vi "Builtin.vi"() -> ()   [LabVIEW 2016]
uses:
  <vilib>/Rock Robotics/WPI/Accelerometer/ADXL345 Range.ctl
  <vilib>/Rock Robotics/SystemInterfaces/spilib/spi_bus.ctl
  <vilib>/Rock Robotics/Network Tables/NT Write Numeric Array.vi
  <vilib>/Rock Robotics/WPI/Accelerometer/InternalAccelerometer/WPI_AccelerometerInternalOpen.vi
  <vilib>/Rock Robotics/WPI/Gyro/WPI_GyroAnalogOpen.vi
panel:
  out "Ang Error":dbl
  out "AR Error":dbl
  out "Ang Flutter":dbl
  out "AR Flutter":dbl
  out "Ang Min":dbl
  out "AR Min":dbl
  out "Ang Max":dbl
  out "AR Max":dbl
  out "Angle":dbl
  out "Angular Rate":dbl
  out "Angle":dbl
  out "Calibrated?":bool
  in  "Reset Gyro?":bool
  out "Gyro Found?":bool
  out "Connection Count":i32
  out "Connected":bool
  out "Z Flut":dbl(graph)
  out "Y Flut":dbl(graph)
  out "X Flut":dbl(graph)
  out "Z Accel":dbl(graph)
  out "Y Accel":dbl(graph)
  out "Z Error":dbl
  out "Y Error":dbl
  out "X Error":dbl
  out "X Accel":dbl(graph)
  out "Z Flutter":dbl
  out "Y Flutter":dbl
  out "X Flutter":dbl
  out "X Min":dbl
  out "Y Min":dbl
  out "Z Min":dbl
  out "X Max":dbl
  out "Y Max":dbl
  out "Z Max":dbl
  in  "Accel Range":T1 items=["+/- 2 g", "+/- 4 g", "+/- 8 g", "+/- 16 g"]
  in  "stop":bool
  out "X Acceleration":dbl
  out "Y Acceleration":dbl
  out "Z Acceleration":dbl
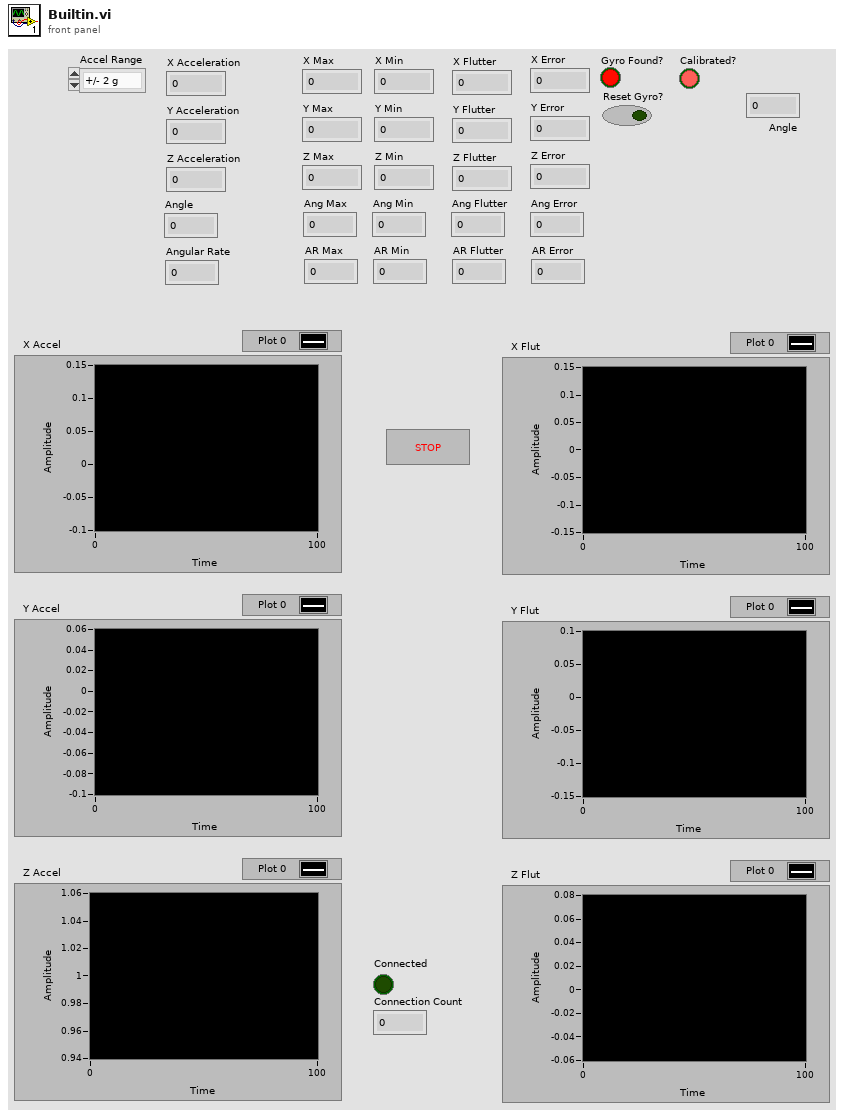
[diagram p1: front panel]
types:
  T1 = typedef "ADXL345 Range.ctl" = u8
  T2 = typedef "spi_bus.ctl" = enum16{"SPI On-Board, CS0", "SPI On-Board, CS1", "SPI On-Board, CS2", "SPI On-Board, CS3", "SPI MXP", "Invalid"}
  T3 = typedef "WPI_GyroDevRef.ctl" = cluster{"DevStatus":errorcluster, "Analog Channel":T4, "Offset":dbl, "Gain (VoltsPerDegree/Second)":dbl, "Gyro Type":enum16{"Analog", "XRS450"}, "Handle":i32, "SPI Bus":T2, "Device Found":bool, "Sample Rate":dbl, "Calibrate On Open":bool}
  T4 = typedef "FPGA_AIChannel.ctl" = enum8{"AI 0", "AI 1", "AI 2", "AI 3", "AI MXP 0", "AI MXP 1", "AI MXP 2", "AI MXP 3", "Invalid"}
  T5 = typedef "WPI_AccelerometerDevRef.ctl" = cluster{"DevStatus":errorcluster, "Scaling":T6, "Analog Channels":T7, "I2C Bus":T8, "SPI Bus":T2, "Accel Range":T1, "ADXL Axes":T9, "Handle":i32, "Device Address":u8, "Accel Type":enum16{"Analog", "ADXL345 I2C", "ADXL345 SPI", "Internal", "ADXL362 SPI"}}
  T6 = typedef "WPI_AccelerometerScaling.ctl" = cluster{"Gain (VoltsPerG)":dbl, "Center Voltage":dbl}
  T7 = typedef "WPI_AccelerometerAnalogChannels.ctl" = cluster{"X-Axis":T4, "Y-Axis":T4, "Z-Axis":T4}
  T8 = typedef "i2c_bus.ctl" = enum16{"I2C On-Board", "I2C MXP", "Invalid"}
  T9 = typedef "WPI_AccelerometerADXL345 Axes.ctl" = cluster{"X-Axis":bool, "Y-Axis":bool, "Z-Axis":bool}
  T10 = cluster{"X-Axis":dbl, "Y-Axis":dbl, "Z-Axis":dbl}
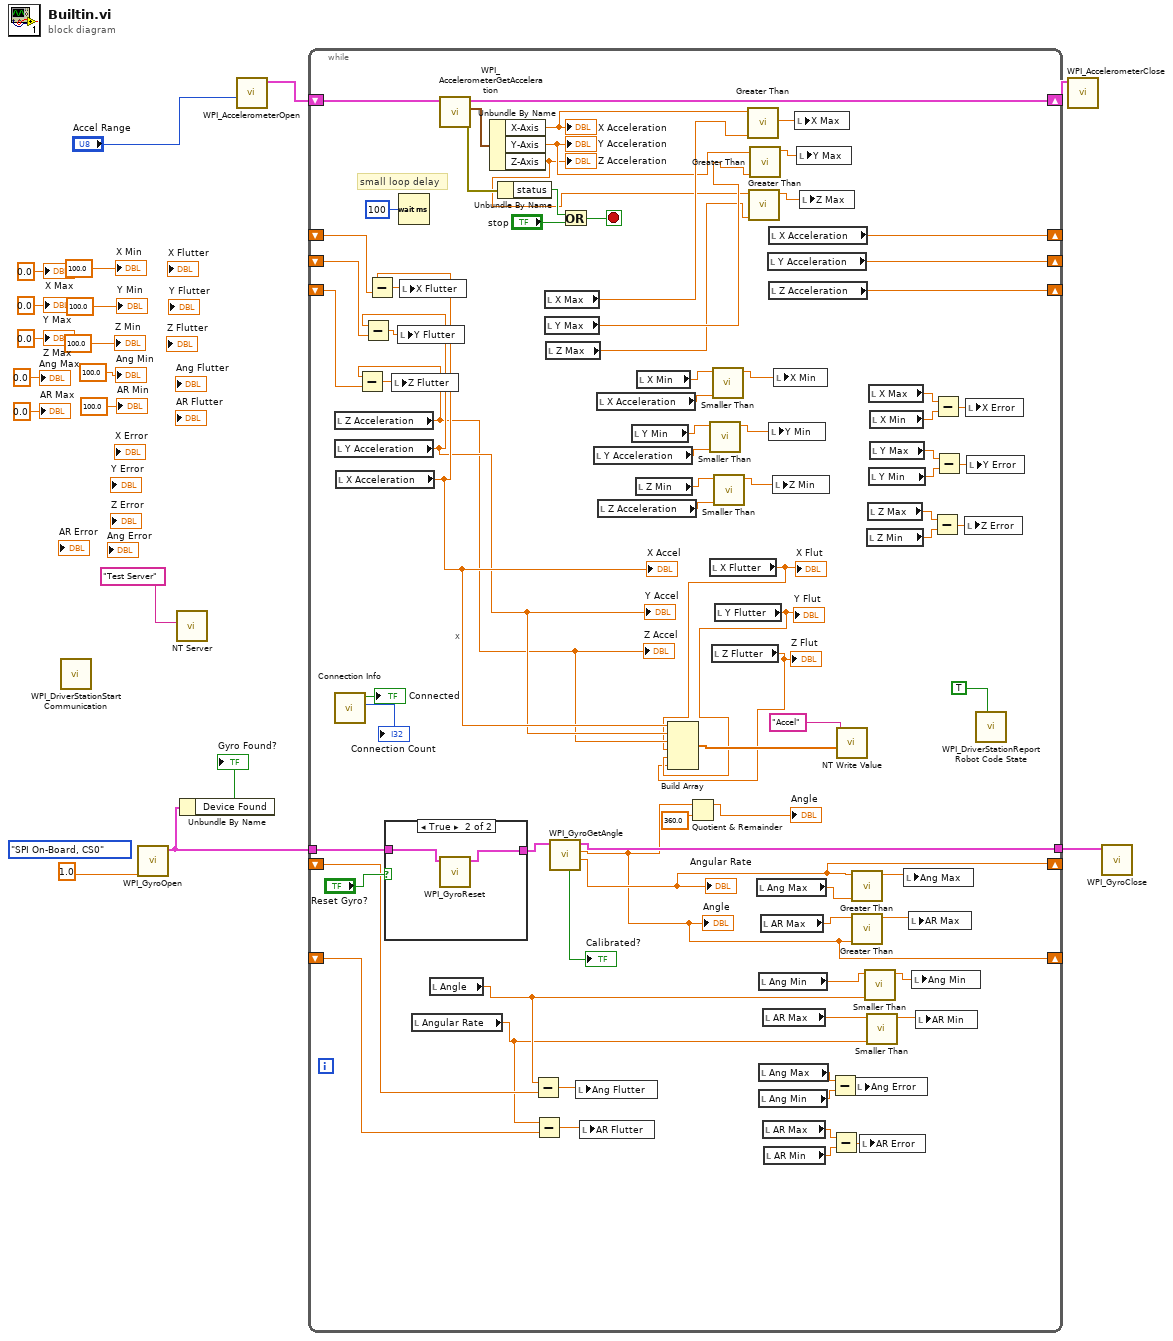
[diagram p0: block diagram]
diagram:
  (unwired) spi_bus."SPI On-Board, CS0" ("SPI Bus")
  n1 = call <vilib>:"WPI_DriverStationStart Communication.vi"() -> ()  [unwired: 12 in]
  n2 = call-poly <vilib>:"WPI_GyroOpen.vi"("Analog Channel"=1.0 ("Sample Rate (ms)")) -> ("GyroDevRef"=w6:T3)  [unwired: 8 in, 2 out]
  n3 = call <vilib>:"NT Server.vi"("Server Name"="Test Server") -> ()  [unwired: 11 in]
  n4 = Unbundle By Name(w6) -> ("Device Found"=→"Gyro Found?":bool)
  n5 = call-poly <vilib>:"WPI_AccelerometerOpen.vi"("Accel Range"="Accel Range") -> ("AccelerometerDevRef"=w18:T5)  [unwired: 9 in, 1 out]
  n6 = while {
    shift-right: [w98] -> w16
    shift-left: w18 -> [w96]
    shift-right: [w76] -> _
    shift-left: _ -> [w71]
    shift-right: [w75] -> _
    shift-left: _ -> [w72]
    shift-right: [w74] -> _
    shift-left: _ -> [w73]
    tunnel: w6 -> [w46]
    tunnel: [w44] -> w5
    shift-right: [w37] -> _
    shift-left: _ -> [w31]
    shift-right: [w36] -> _
    shift-left: _ -> [w27]
    stop <- w97 stop-if-true
    # "X"
    # "small loop delay"
    n7 = local read "Z Acceleration"() -> (w52:dbl)
    "Z Accel" <- w52
    n8 = local read "Y Acceleration"() -> (w53:dbl)
    "Y Accel" <- w53
    n9 = call <vilib>:"Connection Info.vi"() -> ("Connection Count"=→"Connection Count":i32, "Connected"=→"Connected":bool)  [unwired: 10 in]
    n10 = local read "X Acceleration"() -> (w54:dbl)
    "X Accel" <- w54
    n11 = Subtract(x=w52, y=w73) -> (x-y=w68:dbl)
    n12 = Subtract(x=w53, y=w72) -> (x-y=w69:dbl)
    n13 = Subtract(x=w54, y=w71) -> (x-y=w70:dbl)
    n14 = case shown="True" "Reset Gyro?" {
      tunnel: w46 -> [w103 w105]
      tunnel: [w103 w104] -> w45
      frame False {
      }
      frame True {
        n15 = call <vilib>:"WPI_GyroReset.vi"("GyroDevRef"=w105) -> ("GyroDevRef"=w104:T3)  [unwired: 9 in, 1 out]
      }
    }
    n16 = local write "Z Flutter"(w68) -> ()
    n17 = local write "Y Flutter"(w69) -> ()
    n18 = Wait (ms)(milliseconds to wait=u32 100) -> ()  [unwired: 1 out]
    n19 = local write "X Flutter"(w70) -> ()
    n20 = local read "Angular Rate"() -> (w26:dbl)
    n21 = local read "Angle"() -> (w30:dbl)
    n22 = call <vilib>:"WPI_AccelerometerGetAcceleration.vi"("AccelerometerDevRef"=w96) -> ("error out"=w95:errorcluster, "Accelerations"=w99:T10, "AccelerometerDevRef"=w98:T5)  [unwired: 8 in]
    n23 = Unbundle By Name(w99) -> ("X-Axis"=w94:dbl, "Y-Axis"=w91:dbl, "Z-Axis"=w88:dbl)
    "X Acceleration" <- w94
    "Y Acceleration" <- w91
    "Z Acceleration" <- w88
    n24 = Unbundle By Name(w95) -> ("status"=w102:bool)
    n25 = Subtract(x=w30, y=w31) -> (x-y=w29:dbl)
    n26 = Subtract(x=w26, y=w27) -> (x-y=w28:dbl)
    n27 = local read "X Max"() -> (w93:dbl)
    n28 = local read "Y Max"() -> (w90:dbl)
    n29 = local read "Z Max"() -> (w87:dbl)
    n30 = call <vilib>:"WPI_GyroGetAngle.vi"("GyroDevRef"=w45) -> ("Angular Rate"=w37:dbl, "Angle"=w36:dbl, "GyroDevRef"=w44:T3, "Calibrated?"=→"Calibrated?":bool)  [unwired: 6 in, 1 out]
    "Angular Rate" <- w37
    "Angle" <- w36
    n31 = Or(x=w102, y="stop") -> (x .or. y?=w97:bool)
    n32 = local write "Ang Flutter"(w29) -> ()
    n33 = local write "AR Flutter"(w28) -> ()
    n34 = local read "Y Acceleration"() -> (w82:dbl)
    n35 = local read "X Acceleration"() -> (w83:dbl)
    n36 = local read "Z Acceleration"() -> (w77:dbl)
    n37 = local read "Y Min"() -> (w81:dbl)
    n38 = local read "Z Min"() -> (w78:dbl)
    n39 = local read "X Min"() -> (w84:dbl)
    n40 = Quotient & Remainder(x=w36, y=360.0) -> (x-y*floor(x/y)=→"Angle":dbl)  [unwired: 1 out]
    n41 = call "Smaller Than.vi"("N2"=w82, "N1"=w81) -> ("Smaller Number"=w80:dbl)  [unwired: 9 in]
    n42 = local read "X Flutter"() -> (w50:dbl)
    "X Flut" <- w50
    n43 = local read "Z Flutter"() -> (w48:dbl)
    "Z Flut" <- w48
    n44 = call "Smaller Than.vi"("N2"=w83, "N1"=w84) -> ("Smaller Number"=w85:dbl)  [unwired: 9 in]
    n45 = call "Smaller Than.vi"("N2"=w77, "N1"=w78) -> ("Smaller Number"=w79:dbl)  [unwired: 9 in]
    n46 = local read "Y Flutter"() -> (w49:dbl)
    "Y Flut" <- w49
    n47 = Build Array(w54, w53, w52, w50, w49, w48) -> (w51:dbl[])
    n48 = call "Greater Than.vi"("N2"=w93, "N1"=w94) -> ("Greater  Number"=w92:dbl)  [unwired: 9 in]
    n49 = call "Greater Than.vi"("N2"=w87, "N1"=w88) -> ("Greater  Number"=w86:dbl)  [unwired: 9 in]
    n50 = call "Greater Than.vi"("N2"=w90, "N1"=w91) -> ("Greater  Number"=w89:dbl)  [unwired: 9 in]
    n51 = local read "Ang Max"() -> (w41:dbl)
    n52 = local read "Ang Min"() -> (w35:dbl)
    n53 = local read "Ang Max"() -> (w20:dbl)
    n54 = local read "Ang Min"() -> (w21:dbl)
    n55 = local read "AR Max"() -> (w39:dbl)
    n56 = local read "AR Max"() -> (w33:dbl)
    n57 = local read "AR Max"() -> (w25:dbl)
    n58 = local read "AR Min"() -> (w24:dbl)
    n59 = local read "Y Acceleration"() -> (w75:dbl)
    n60 = local read "X Acceleration"() -> (w76:dbl)
    n61 = local read "Z Acceleration"() -> (w74:dbl)
    n62 = local write "Y Min"(w80) -> ()
    n63 = local write "Z Min"(w79) -> ()
    n64 = local write "X Min"(w85) -> ()
    n65 = local write "X Max"(w92) -> ()
    n66 = local write "Y Max"(w89) -> ()
    n67 = local write "Z Max"(w86) -> ()
    n68 = Subtract(x=w20, y=w21) -> (x-y=w22:dbl)
    n69 = Subtract(x=w25, y=w24) -> (x-y=w23:dbl)
    n70 = call-poly <vilib>:"NT Write Value.vi"("Numeric Array"=w51, "Name"="Accel") -> ()  [unwired: 9 in, 1 out]
    n71 = call "Greater Than.vi"("N2"=w41, "N1"=w37) -> ("Greater  Number"=w40:dbl)  [unwired: 9 in]
    n72 = call "Greater Than.vi"("N2"=w36, "N1"=w39) -> ("Greater  Number"=w38:dbl)  [unwired: 9 in]
    n73 = local write "Ang Error"(w22) -> ()
    n74 = local write "AR Error"(w23) -> ()
    n75 = call "Smaller Than.vi"("N2"=w30, "N1"=w35) -> ("Smaller Number"=w34:dbl)  [unwired: 9 in]
    n76 = local read "Z Min"() -> (w60:dbl)
    n77 = call "Smaller Than.vi"("N2"=w26, "N1"=w33) -> ("Smaller Number"=w32:dbl)  [unwired: 9 in]
    n78 = local read "Z Max"() -> (w61:dbl)
    n79 = local read "X Max"() -> (w67:dbl)
    n80 = local read "Y Min"() -> (w63:dbl)
    n81 = local read "X Min"() -> (w66:dbl)
    n82 = local read "Y Max"() -> (w62:dbl)
    n83 = local write "Ang Max"(w40) -> ()
    n84 = local write "AR Max"(w38) -> ()
    n85 = local write "Ang Min"(w34) -> ()
    n86 = local write "AR Min"(w32) -> ()
    n87 = Subtract(x=w61, y=w60) -> (x-y=w59:dbl)
    n88 = Subtract(x=w67, y=w66) -> (x-y=w65:dbl)
    n89 = Subtract(x=w62, y=w63) -> (x-y=w64:dbl)
    n90 = local write "Z Error"(w59) -> ()
    n91 = local write "X Error"(w65) -> ()
    n92 = local write "Y Error"(w64) -> ()
    n93 = call <vilib>:"WPI_DriverStationReport Robot Code State.vi"("Test"=TRUE) -> ()  [unwired: 10 in, 1 out]
  }
  n94 = call <vilib>:"WPI_AccelerometerClose.vi"("AccelerometerDevRef"=w16) -> ()  [unwired: 10 in, 1 out]
  n95 = call <vilib>:"WPI_GyroClose.vi"("GyroDevRef"=w5) -> ()  [unwired: 10 in, 1 out]
  "Z Max" <- 0.0 ("Z Max")
  "Y Max" <- 0.0 ("Y Max")
  "X Max" <- 0.0 ("X Max")
  "Z Min" <- 100.0 ("Z Min")
  "Y Min" <- 100.0 ("Y Min")
  "X Min" <- 100.0 ("X Min")
  "AR Max" <- 0.0 ("AR Max")
  "Ang Max" <- 0.0 ("Ang Max")
  "AR Min" <- 100.0 ("AR Min")
  "Ang Min" <- 100.0 ("Ang Min")
